vi "程序设置-加载列表.vi"() -> (0 "error out":errorcluster, 3 "文件名显示":string[](array[string]))   [LabVIEW 2017]
uses:
  <vilib>/Utility/xml.llb/Read From XML File(array).vi
panel:
  out "程序注释信息":string
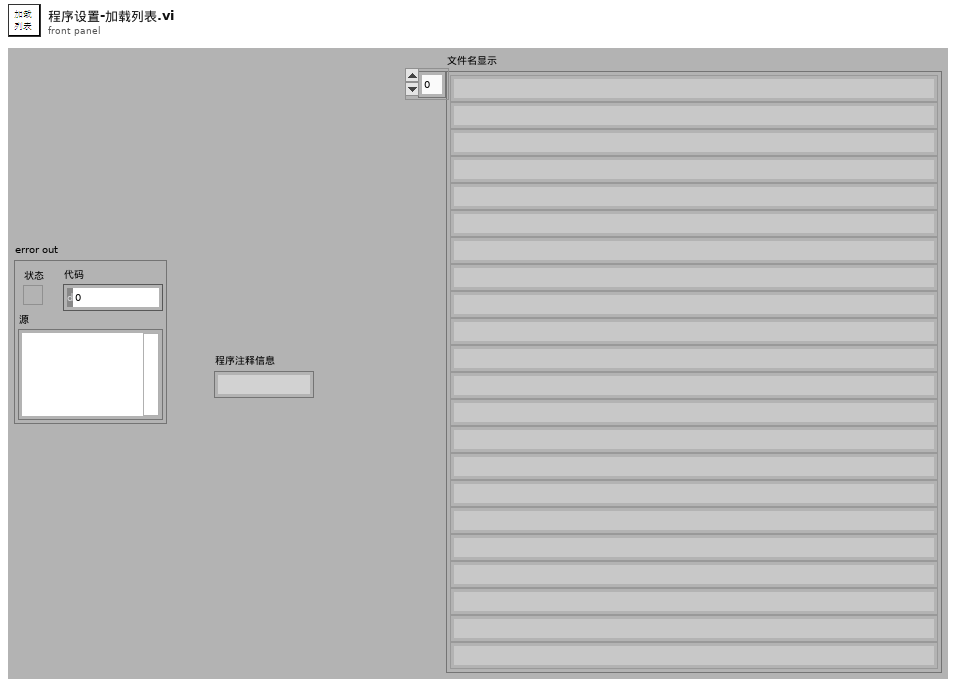
[diagram p1: front panel]
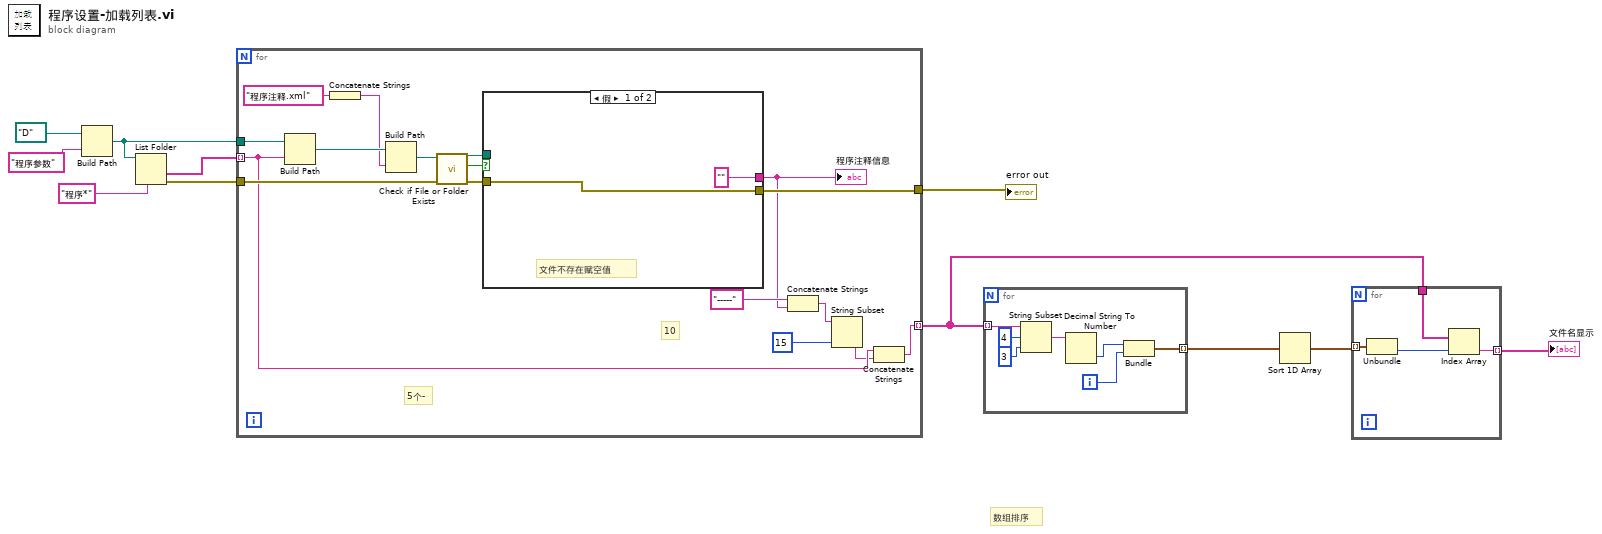
[diagram p0: block diagram]
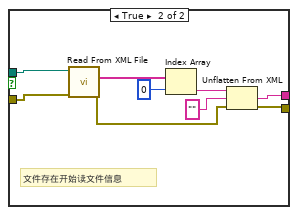
[diagram p2: hidden frame]
diagram:
  # "数组排序"
  n1 = Build Path(base path=path "D:/" ("基路径"), name or relative path="程序参数" ("名称或相对路径")) -> (appended path=w7:path)
  n2 = List Folder(path=w7, pattern="程序*" ("模式")) -> (folder names=w9:string[], error out=w8:errorcluster)  [unwired: 2 in, 2 out]
  n3 = for {
    tunnel: w9 -> [w17] mode=indexing
    tunnel: w7 -> [w28]
    tunnel: w8 -> [w21]
    tunnel: [w22] -> w6
    tunnel: [w18] -> w4 mode=indexing
    # "10"
    # "5个-"
    n4 = Build Path(base path=w28, name or relative path=w17) -> (appended path=w27:path)
    n5 = Concatenate Strings("程序注释.xml" ("名称或相对路径")) -> (w12:string)
    n6 = Build Path(base path=w27, name or relative path=w12) -> (appended path=w26:path)
    n7 = call <vilib>:"Check if File or Folder Exists.vi"("error in (no error)"=w21, "path"=w26) -> ("error out"=w23:errorcluster, "file or folder exists?"=w25:bool, "dup path"=w24:path)  [unwired: 7 in]
    n8 = case shown="假" w25 {
      tunnel: w24 -> [_ w39]
      tunnel: w23 -> [w29 w31]
      tunnel: ["" ("程序注释信息") w34] -> w14
      tunnel: [w29 w33] -> w22
      frame False {
        # "文件不存在赋空值"
      }
      frame True {
        # "文件存在开始读文件信息"
        n9 = call-poly <vilib>:"Read From XML File.vi"("error in (no error)"=w31, "XML File Path"=w39) -> ("error out"=w32:errorcluster, "XML Elements"=w38:string[])  [unwired: 7 in, 1 out]
        n10 = Index Array(array=w38, index=0 ("索引")) -> (element=w36:string)
        n11 = Unflatten From XML(xml string=w36, type="" ("程序注释信息"), error in (no error)=w32) -> (value=w34:string, error out=w33:errorcluster)
      }
    }
    "程序注释信息" <- w14
    n12 = Concatenate Strings("-----" ("字符串"), w14) -> (w19:string)
    n13 = String Subset(string=w19, length (rest)=15 ("长度（剩余）")) -> (substring=w16:string)  [unwired: 1 in]
    n14 = Concatenate Strings(w17, w16) -> (w18:string)
  }
  "error out" <- w6
  n15 = for {
    tunnel: w4 -> [w45] mode=indexing
    tunnel: [w42] -> w3 mode=indexing
    i -> [w46]
    n16 = String Subset(string=w45, offset (0)=4 ("偏移量(0)"), length (rest)=3 ("长度（剩余）")) -> (substring=w41:string)
    n17 = Decimal String To Number(string=w41) -> (number=w40:i32)  [unwired: 2 in, 1 out]
    n18 = Bundle(w40, w46) -> (w42:cluster{i32, i32})  [unwired: 1 in]
  }
  n19 = Sort 1D Array(array=w3) -> (sorted array=w2:cluster{i32, i32}[])
  n20 = for {
    tunnel: w2 -> [w50] mode=indexing
    tunnel: w4 -> [w48]
    tunnel: [w47] -> w5 mode=indexing
    n21 = Unbundle(w50) -> (w49:i32)  [unwired: 1 out]
    n22 = Index Array(array=w48, index=w49) -> (element=w47:string)
  }
  "文件名显示" <- w5
